vi "CarWashUITest.vi"() -> ()   [LabVIEW 2016]
uses:
  Car Wash 16.0/Car Wash.vi
  main/apis/Stimulus/ValueSignalByPathString.vi
  <vilib>/addons/_JKI Toolkits/Caraya/classes/Test/Test.lvclass
  Car Wash 16.0/Car Wash.lvlib
panel:
  out "error out":errorcluster
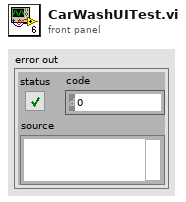
[diagram p1: front panel]
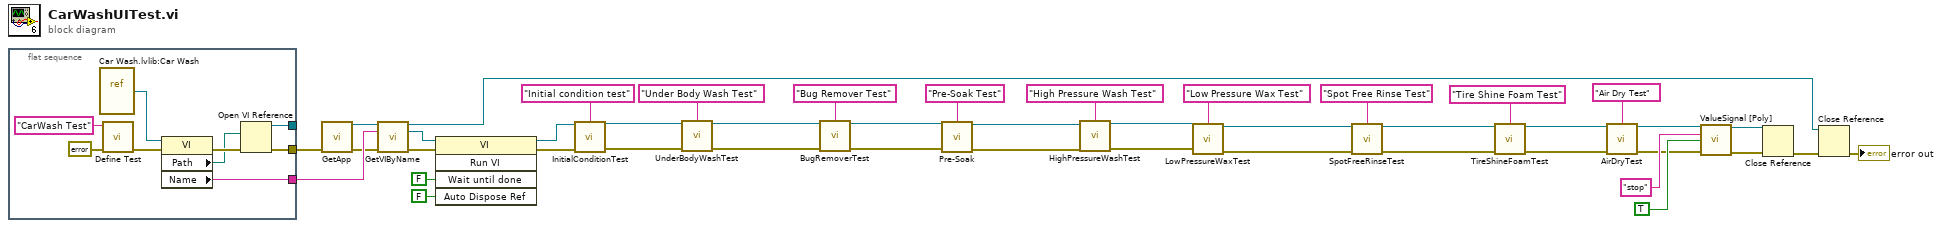
[diagram p0: block diagram]
diagram:
  n1 = flat-sequence {
    tunnel: [w49] -> w43
    tunnel: [w48] -> _
    tunnel: [w46] -> w42
    frame #0 {
      n2 = vi-ref "Car Wash.lvlib:Car Wash.vi"() -> (w51:refnum<vi>)
      n3 = call <vilib>:"Define Test.vi"("error in (no error)"=errorcluster {"status"=FALSE, "code"=0, "source"=""}, "Label (VI Title)"="CarWash Test") -> ("error out"=w52:errorcluster)  [unwired: 9 in]
      n4 = property on="Property Node" class="VI"(reference=w51, error in=w52) -> (error out=w50:errorcluster, "Path"=w47:path, "Name"=w46:string)  [unwired: 1 out]
      n5 = Open VI Reference(vi path=w47, error in (no error)=w50) -> (vi reference=w48:refnum<vi>, error out=w49:errorcluster)  [unwired: 4 in]
    }
  }
  n6 = call "GetApp.vi"("error in (no error)"=w43) -> ("Application Ref"=w44:refnum<vi>, "error out"=w41:errorcluster)  [unwired: 13 in]
  n7 = call "GetVIByName.vi"("Application Ref in"=w44, "VI Name"=w42, "error in (no error)"=w41) -> ("Application Ref out"=w1:refnum<vi>, "VI Reference"=w39:refnum<vi>, "error out"=w40:errorcluster)  [unwired: 10 in]
  n8 = invoke on="Invoke Node" class="VI" method="Run VI"(reference=w39, error in=w40, "Wait until done"=FALSE ("Wait Until Done"), "Auto Dispose Ref"=FALSE ("Auto Dispose Reference")) -> (reference out=w35:refnum<vi>, error out=w36:errorcluster)  [unwired: 1 in, 3 out]
  n9 = call "InitialConditionTest.vi"("VI Reference In"=w35, "Label"="Initial condition test", "error out"=w36) -> ("VI Reference Out"=w32:refnum<vi>, "error out"=w31:errorcluster)  [unwired: 11 in]
  n10 = call "UnderBodyWashTest.vi"("VI Reference In"=w32, "Label"="Under Body Wash Test", "error in"=w31) -> ("VI Reference Out"=w29:refnum<vi>, "error out"=w30:errorcluster)  [unwired: 11 in]
  n11 = call "BugRemoverTest.vi"("VI Reference In"=w29, "Label"="Bug Remover Test", "error in"=w30) -> ("VI Reference Out"=w26:refnum<vi>, "error out"=w27:errorcluster)  [unwired: 11 in]
  n12 = call "Pre-Soak.vi"("VI Reference In"=w26, "Label"="Pre-Soak Test", "error in"=w27) -> ("VI Reference Out"=w23:refnum<vi>, "error out"=w24:errorcluster)  [unwired: 11 in]
  n13 = call "HighPressureWashTest.vi"("VI Reference In"=w23, "Label"="High Pressure Wash Test", "error in"=w24) -> ("VI Reference Out"=w20:refnum<vi>, "error out"=w21:errorcluster)  [unwired: 11 in]
  n14 = call "LowPressureWaxTest.vi"("VI Reference In"=w20, "Label"="Low Pressure Wax Test", "error in"=w21) -> ("VI Reference Out"=w17:refnum<vi>, "error out"=w18:errorcluster)  [unwired: 11 in]
  n15 = call "SpotFreeRinseTest.vi"("VI Reference In"=w17, "Label"="Spot Free Rinse Test", "error in"=w18) -> ("VI Reference Out"=w14:refnum<vi>, "error out"=w15:errorcluster)  [unwired: 11 in]
  n16 = call "TireShineFoamTest.vi"("VI Reference In"=w14, "Label"="Tire Shine Foam Test", "error in"=w15) -> ("VI Reference Out"=w12:refnum<vi>, "error out"=w11:errorcluster)  [unwired: 11 in]
  n17 = call "AirDryTest.vi"("VI Reference In"=w12, "Label"="Air Dry Test", "error in"=w11) -> ("VI Reference Out"=w3:refnum<vi>, "error out"=w4:errorcluster)  [unwired: 11 in]
  n18 = call-poly "ValueSignal [Poly].vi"("VI Reference In"=w3, "Control Name"="stop", "Value (Signaling)"=TRUE, "error in"=w4) -> ("VI Reference Out"=w2:refnum<vi>, "error out"=w7:errorcluster)  [unwired: 10 in]
  n19 = Close Reference(reference=w2, error in (no error)=w7) -> (error out=w6:errorcluster)
  n20 = Close Reference(reference=w1, error in (no error)=w6) -> (error out=→"error out":errorcluster)
